vi "Process.vi"(9 "process sync":refnum<notifier>, 11 "DbgTimers in":refnum<class "DbgTimers.lvclass">) -> ()   [LabVIEW 2017, in "DbgTimers.lvclass"]
doc: "Developed by Kevin Thompson\nkevin@thompsonengineering.net\n\nCopyright 2018-2020\nThompson Engineering, LLC"
uses:
  DbgTimers.lvclass
  DataTypes/Read Data--cluster.ctl
  DataTypes/Process - AppData--cluster.ctl
  DataTypes/Settings--cluster.ctl
  DataTypes/Dependency--cluster.ctl
  DataTypes/Public Events--cluster.ctl
  Ichor_Common/DataTypes/TD Async CmdMsg EventData--cluster.ctl
  DbgTimers.lvclass/DbgTimers.ctl
  DataTypes/AsynMsg_DbgTimers--enum.ctl
  Accessors/Get Settings.vi
  Accessors/Get PublicEvents.vi
  Accessors/Get Dependency.vi
  Accessors/Get ObjData.vi
  Accessors/Set ObjData.vi
  <vilib>/TELLC/SMQ/Add States to Queue using MultiLine String with vData.vi
  Ichor_Common/Lib/ErrorHandler/ErrorHandler.lvclass
panel:
  out "LogFile path":path
  in  "Enable msTick Logging":bool
  out "DbgTimersReadData":T1
  in  "Exit":bool
  # "local data monitoring"
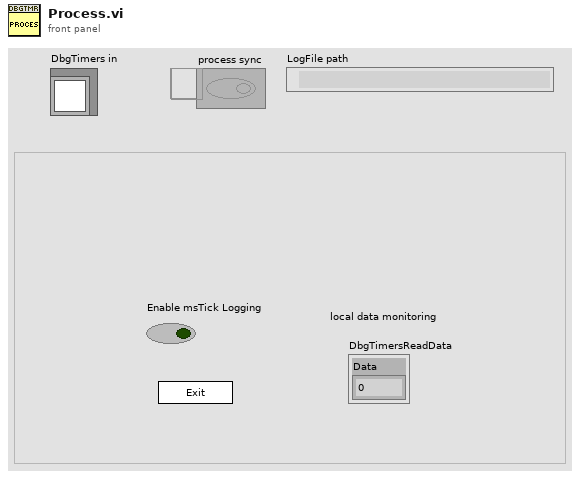
[diagram p1: front panel]
types:
  T1 = typedef "DbgTimers.lvclass/Read Data--cluster.ctl" = cluster{"Data":dbl}
  T2 = typedef "DbgTimers.lvclass/Process - AppData--cluster.ctl" = cluster{"Core":cluster{"Current VI Reference":refnum<vi>, "Close Panel on Exit?":bool}, "Your Boolean data":bool, "Your string data":string, "SMQ":refnum<queue>, "Initialized?":bool, "Self Reference":refnum<class "DbgTimers.lvclass">, "Simulation?":bool, "process sync":refnum<notifier>, "vData":variant, "Settings":T3, "Dependency":T4, "Public Events":T5, "msTickLogging?":bool}
  T3 = typedef "DbgTimers.lvclass/Settings--cluster.ctl" = cluster{"Simulation":bool, "DbgTimer LogFolder":path}
  T4 = typedef "DbgTimers.lvclass/Dependency--cluster.ctl" = cluster{"Config":refnum<class>, "ClassRef":refnum<class>}
  T5 = typedef "DbgTimers.lvclass/Public Events--cluster.ctl" = cluster{"DbgTimers.AsyncCmd Event":refnum<user-event>, "DbgTimers.AsyncMsg Event":refnum<user-event>, "stop process":refnum<user-event>}
  T6 = typedef "TELLC_Temp01.lvclass/Dependency--cluster.ctl" = cluster{"Config":refnum<class>, "ClassRef":refnum<class>}
  T7 = typedef "DbgTimers.lvclass/AsynMsg_DbgTimers--enum.ctl" = enum16{"DbgTimers.msTickLogEnabled"}
  T8 = enum32{"invalid app kind", "Development System", "Run Time System", "Student Edition", "Embedded LabVIEW", "Evaluation", "Custom"}
  T9 = enum32{"Invalid", "Standard", "Closed", "Hidden", "Minimized", "Maximized"}
  T10 = typedef "DbgTimers.lvclass/AsynCmd_DbgTimers--enum.ctl" = enum16{"DbgTimers.EnMsTickLogging", "DbgTimers.SetLogFolder"}
  T11 = typedef "DbgTimers.lvclass/ObjData--cluster.ctl" = cluster{"Settings":T3, "ReadData-placeholder":T1, "Timers":T12, "Enable msTick Logging":bool, "LogFile_msTickTimer":path}
  T12 = typedef "DbgTimers.lvclass/Timers--cluster.ctl" = cluster{"ms tick timers":T13[]}
  T13 = typedef "DbgTimers.lvclass/Millisecond Tick Timer--cluster.ctl" = cluster{"startTick":u32, "currentTick":u32, "elapsedTicks":u32, "totalElapsedTicks":u32}
  T14 = cluster{"Current VI Reference":refnum<vi>, "Close Panel on Exit?":bool}
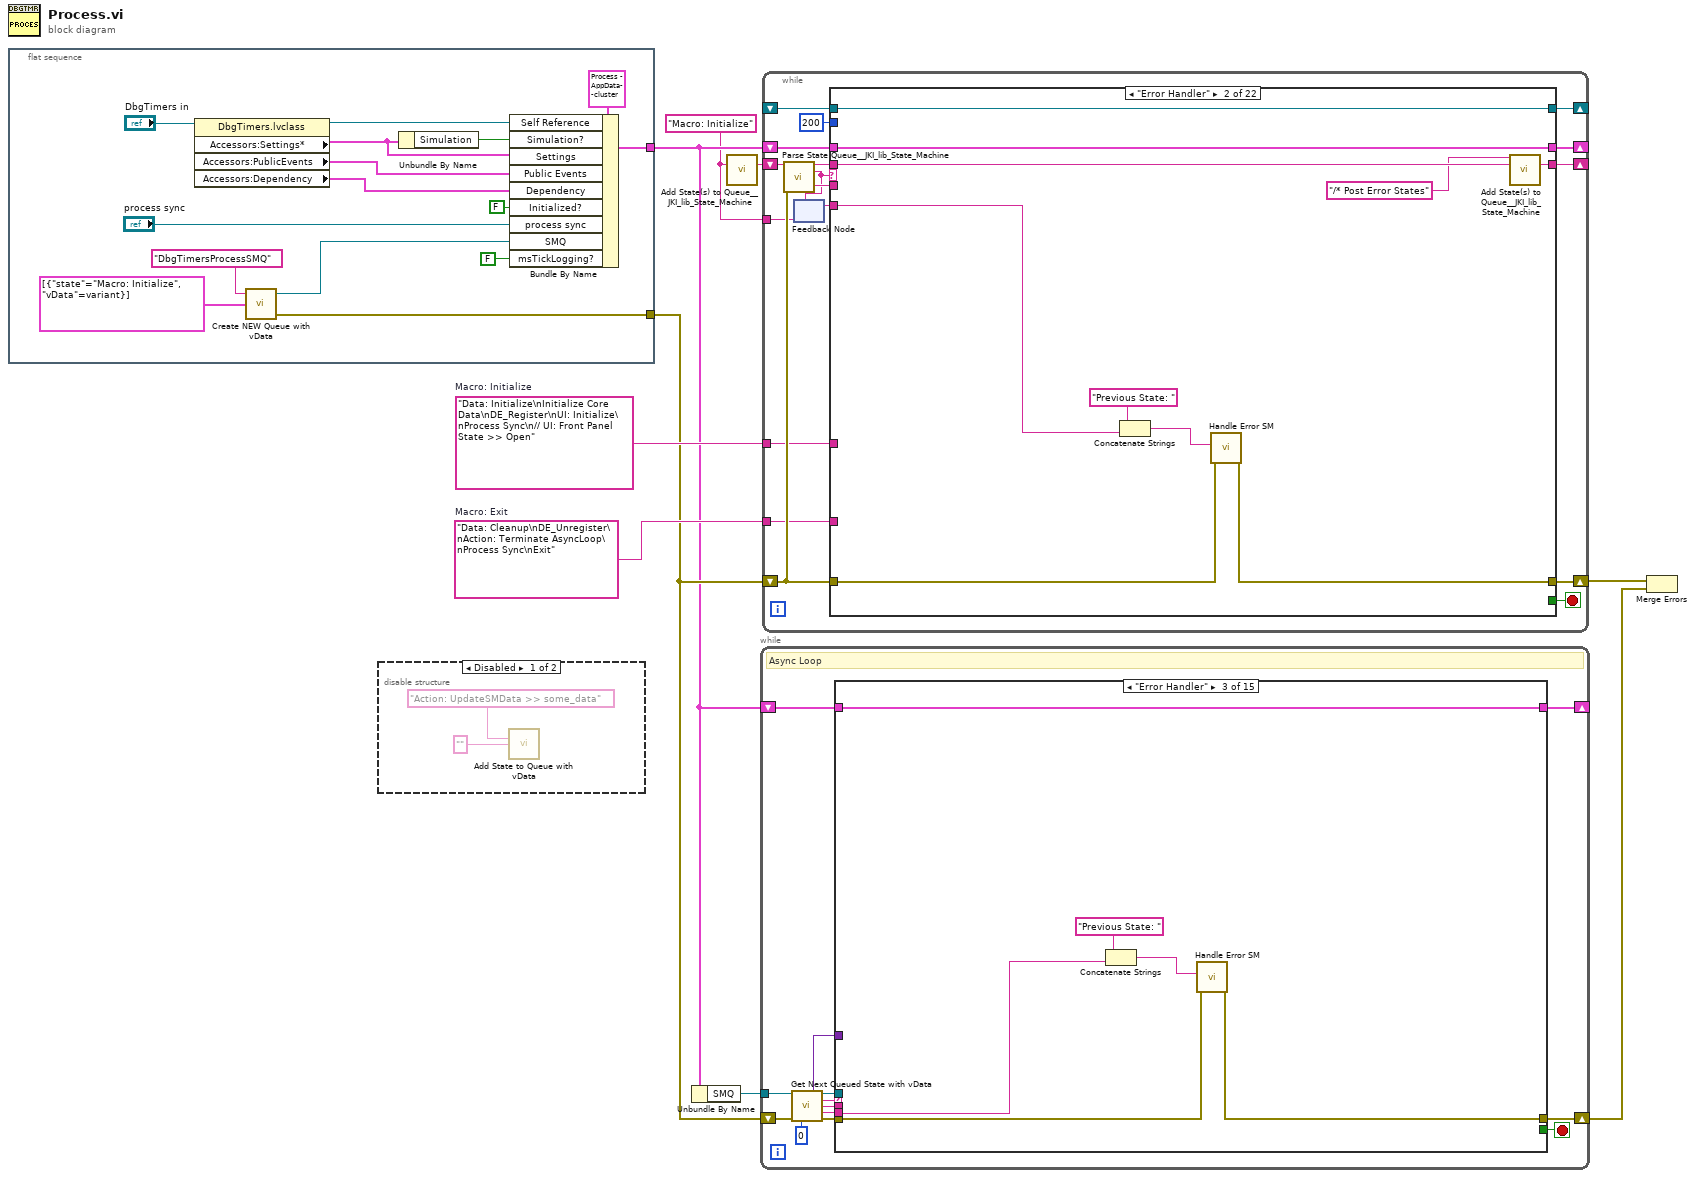
[diagram p0: block diagram]
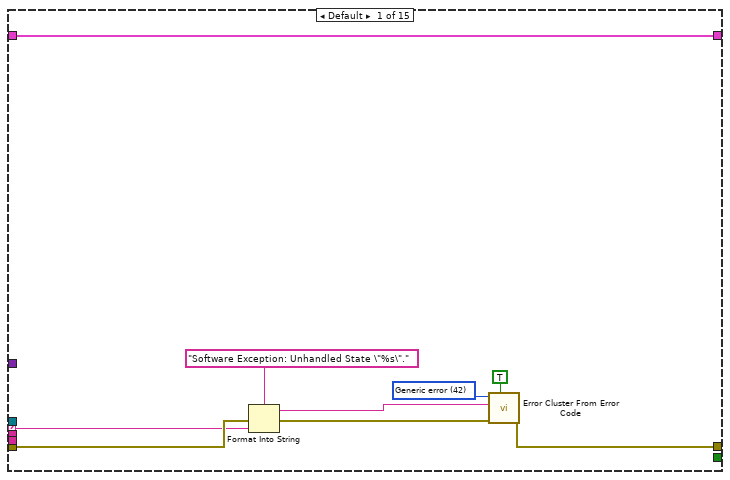
[diagram p3: hidden frame]
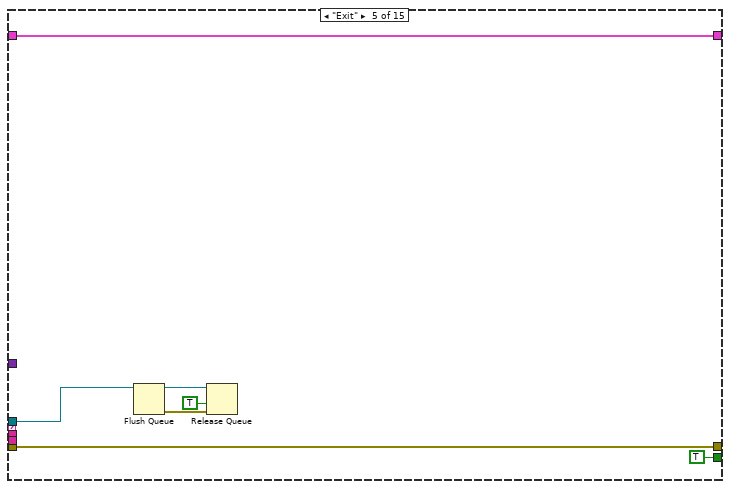
[diagram p6: hidden frame]
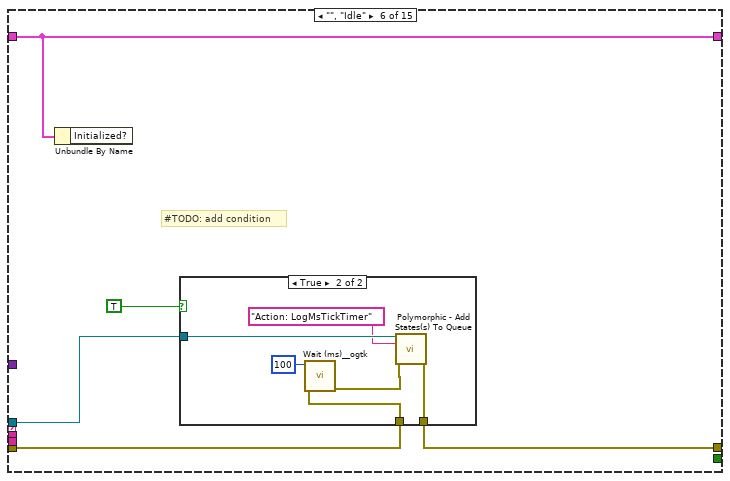
[diagram p7: hidden frame]
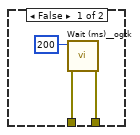
[diagram p8: hidden frame]
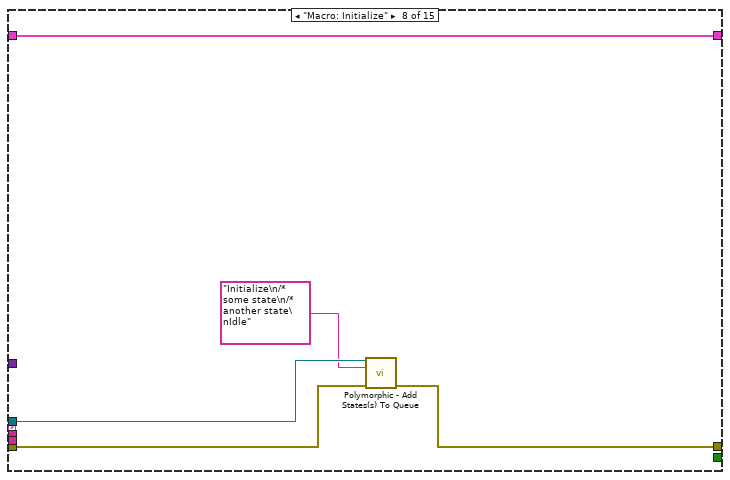
[diagram p10: hidden frame]
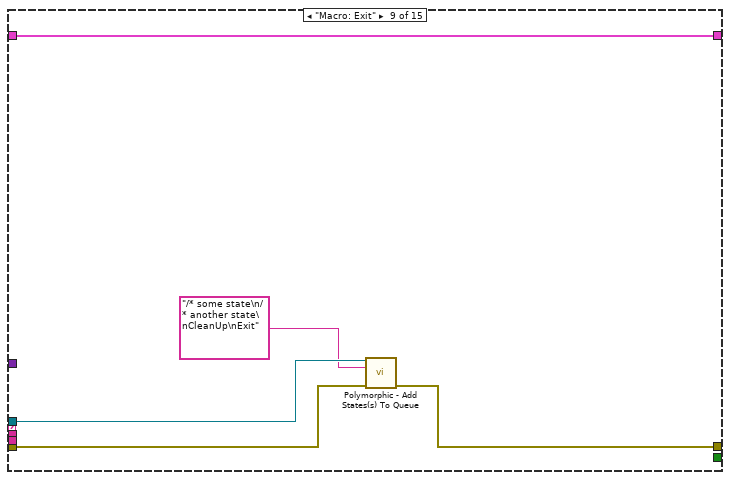
[diagram p11: hidden frame]
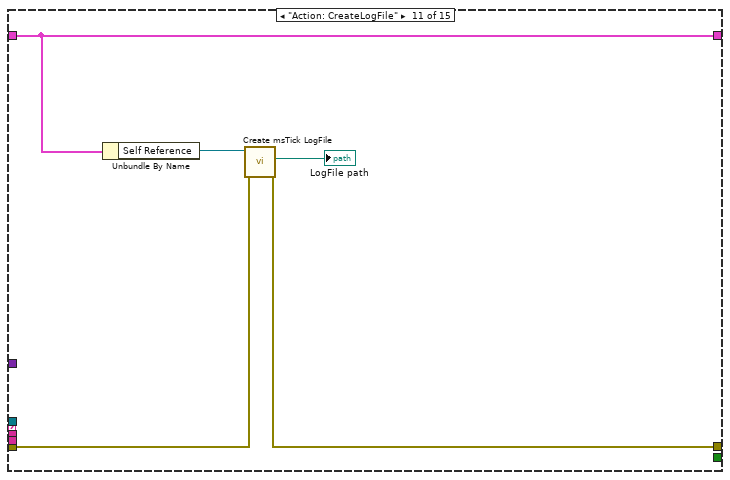
[diagram p13: hidden frame]
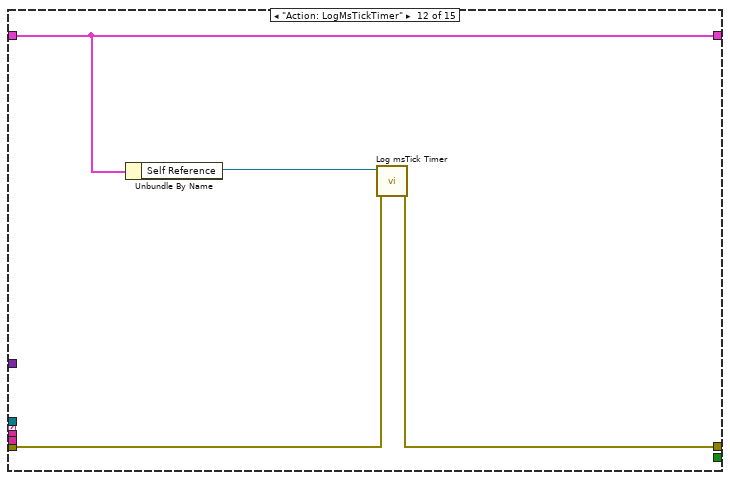
[diagram p14: hidden frame]
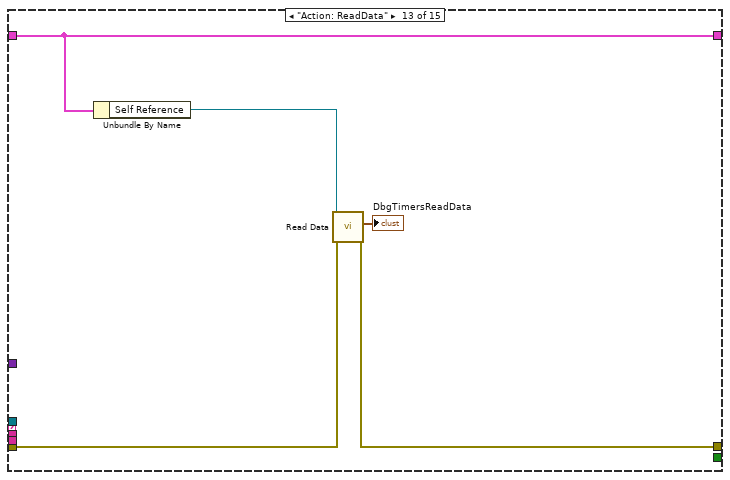
[diagram p15: hidden frame]
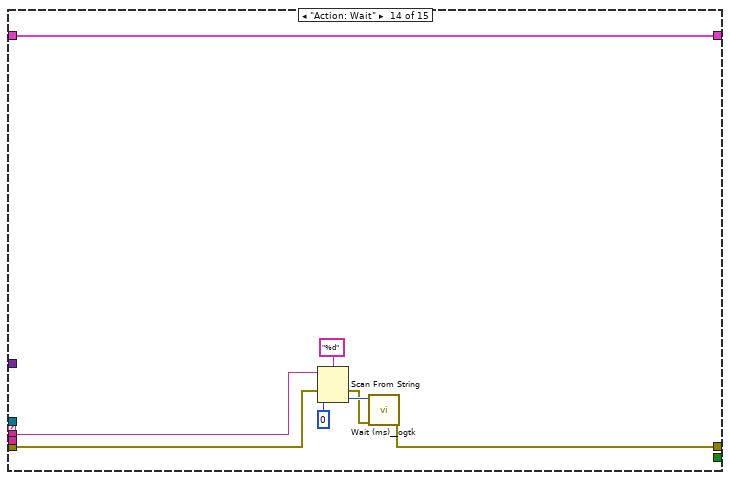
[diagram p16: hidden frame]
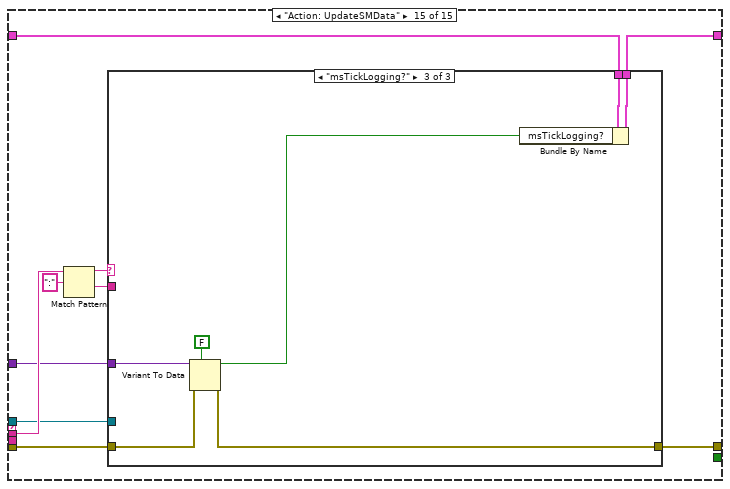
[diagram p17: hidden frame]
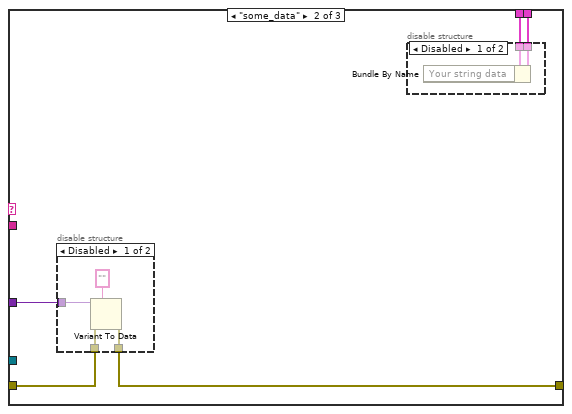
[diagram p19: hidden frame]
diagram:
  w7 = "Data: Cleanup\nDE_Unregister\nAction: Terminate AsyncLoop\nProcess Sync\nExit"  # Macro: Exit
  w8 = "Data: Initialize\nInitialize Core Data\nDE_Register\nUI: Initialize\nProcess Sync\n// UI: Front Panel State >> Open"  # Macro: Initialize
  w1 = "Macro: Initialize"
  n1 = flat-sequence {
    tunnel: [w24] -> w4
    tunnel: [w21] -> w6
    frame #0 {
      n2 = property class="DbgTimers.lvclass"(reference="DbgTimers in") -> (reference out=w17:refnum<class "DbgTimers.lvclass">, "Accessors:Settings*"=w12:T3, "Accessors:PublicEvents"=w14:T5, "Accessors:Dependency"=w15:T6)  [unwired: 1 in, 1 out]
      n3 = call <vilib>:"Create NEW Queue with vData.vi"("Initial States"=cluster{"state":string, "vData":variant}[] [{"state"="Macro: Initialize", "vData"=variant}], "Name (SMQ)"="DbgTimersProcessSMQ") -> ("error out"=w21:errorcluster, "queue out"=w23:refnum<queue>)  [unwired: 2 in]
      n4 = Unbundle By Name(w12) -> ("Simulation"=w13:bool)
      n5 = Bundle By Name(cluster=T2 {"Core"={"Current VI Reference"=refnum, "Close Panel on Exit?"=FALSE}, "Your Boolean data"=FALSE, "Your string data"="", "SMQ"=refnum, "Initialized?"=FALSE, "Self Reference"=refnum, "Simulation?"=FALSE, "process sync"=refnum, "vData"=variant, "Settings"={"Simulation"=FALSE, "DbgTimer LogFolder"=path ""}, "Dependency"={"Config"=refnum, "ClassRef"=refnum}, "Public Events"={"DbgTimers.AsyncCmd Event"=refnum, "DbgTimers.AsyncMsg Event"=refnum, "stop process"=refnum}, "msTickLogging?"=FALSE} ("SM2 AppData"), "Self Reference"=w17, "Simulation?"=w13, "Settings"=w12, "Public Events"=w14, "Dependency"=w15, "Initialized?"=FALSE, "process sync"="process sync", "SMQ"=w23, "msTickLogging?"=FALSE) -> (w24:T2)
    }
  }
  n6 = disable-structure shown="Disabled" {
    frame Disabled {
      n7 = call <vilib>:"Add State to Queue with vData.vi"("state in"="Action: UpdateSMData >> some_data", "vData (\"\")"="") -> ()  [unwired: 10 in, 4 out]
    }
    frame Enabled {
    }
  }
  n8 = Unbundle By Name(w4) -> ("SMQ"=w5:refnum<queue>)
  n9 = call <vilib>:"Add State(s) to Queue__JKI_lib_State_Machine.vi"("State(s) in (\"\")"=w1) -> ("States Out"=w9:string)  [unwired: 14 in]
  n10 = while {
    shift-right: [w36] -> w2
    shift-left: w6 -> [w38]
    tunnel: w5 -> [w34]
    shift-right: [w32] -> _
    shift-left: w4 -> [w33]
    stop <- w27 stop-if-true
    # "Async Loop"
    n11 = call <vilib>:"Get Next Queued State with vData.vi"("queue in"=w34, "error in (no error)"=w38, "timeout (100)"=0) -> ("vData out"=w31:variant, "queue out"=w35:refnum<queue>, "Next State"=w39:string, "queued msg"=w29:string, "Prev State"=w28:string, "error out"=w37:errorcluster)  [unwired: 6 in, 1 out]
    n12 = case shown="\"Error Handler\"" w39 {
      tunnel: w35 -> [_ _ _ _ w59 w67 _ w85 w90 _ _ _ _ _ w121]
      tunnel: w29 -> [_ _ _ _ _ _ _ _ _ _ _ _ _ w110 w123]
      selector: w39 -> [w40 _ _ _ _ _ _ _ _ _ _ _ _ _ _]
      tunnel: w37 -> [w42 w50 w53 w58 w65 w70 w81 w84 w89 w93 w96 w100 w105 w109 w118]
      tunnel: [w41 w50 w52 w58 w65 w69 w81 w83 w88 w93 w95 w99 w104 w112 w117] -> w36
      tunnel: w33 -> [w48 w49 w56 w57 w64 w66 w80 w86 w91 w92 w98 w102 w107 w115 w120]
      tunnel: [w48 w49 w56 w57 w64 w66 w80 w86 w91 w92 w98 w102 w107 w115 w119] -> w32
      tunnel: w31 -> [_ _ _ _ _ _ _ _ _ _ _ _ _ _ w122]
      tunnel: w28 -> [_ _ w51 _ _ _ _ _ _ _ _ _ _ _ _]
      tunnel: [_ _ _ _ TRUE _ _ _ _ _ _ _ _ _ _] -> w27
      frame Default {
        w44 = 42 items=["No error", "Argument error", "Memory is full", "Out of zone", "End of file", "File already open", "Generic file I/O error", "File not found", "File permission error", "Disk is full", "Duplicate path", "Too many files open", "System feature not enabled", "Resource file not found", "Cannot add resource", "Resource not found", "Image not found", "Image memory error", "Pen does not exist", "Config type invalid", "Config token not found", "Config parse error", "Config memory error", "Bad external code format", "Bad external code offset", "External code not present", "Null window", "Destroy window error", "Null menu", "Print aborted", "Bad print record", "Print driver error", "Windows error during printing", "Memory error during printing", "Print dialog error", "Generic print error", "Invalid device refnum", "Device not found", "Device parameter error", "Device unit error", "Cannot open device", "Device call aborted", "Generic error", "Cancelled by user", "Object ID too low", "Object ID too high", "Object not in heap", "Unknown heap", "Unknown object (invalid DefProc)", "Unknown object (DefProc not in table)", "Message out of range", "Invalid (null) method", "Unknown message", "Manager call not supported", "Bad address", "Network operation in progress", "Network operation timed out", "Connection is busy", "Network attribute not supported", "Network error", "Address in use", "System out of memory", "Connection aborted", "Connection refused", "Not connected", "Already connected", "Connection closed", "Initialization error (interapplication manager)", "Bad occurrence", "Wait on unbound occurrence handler", "Occurrence queue overflow", "Datalog type conflict", "Unused", "Unrecognized type (interapplication manager)", "Memory corrupt", "Failed to make temporary DLL", "Old CIN version", "Drag socket not found", "Failed to load drop-object", "Failed to register OLE object", "Failed to release OLE object", "Format specifier type mismatch", "Unknown format specifier", "Too few format specifiers", "Too many format specifiers", "Scan failed", "Newer CIN version", "Error converting to variant", "Runtime menu error", "Password tampered", "Variant attribute not found", "Incompatible variant data type", "Event data is not available", "Event Store is not present", "Occurrence is not found", "Event Queue is not created", "Event info is not available", "Refnum passed is NULL", "Error retrieving Class GUID", "Error retrieving CoClass GUID", "Error retrieving TypeLib GUID.", "Bad built application magic bytes.", "Specific driver is different from the specific driver associated with the Logical Name.", "There is no session opened to the class driver.", "Max Error", "MAX - Error with config objects", "MAX - Error loading configuration", "MAX - Group not supported"]
        n13 = Format Into String(format string="Software Exception: Unhandled State \"%s\"." ("message"), error in=w42, w40) -> (resulting string=w45:string, error out=w46:errorcluster)  [unwired: 1 in]
        n14 = call <vilib>:"Error Cluster From Error Code.vi"("show call chain? (False)"=TRUE, "error in (no error)"=w46, "error message (\"\")"=w45, "error code (0)"=w44) -> ("error out"=w41:errorcluster)  [unwired: 5 in]
      }
      frame "Initialize" {
      }
      frame "Error Handler" {
        n15 = Concatenate Strings("Previous State: ", w51) -> (w54:string)
        n16 = call "Handle Error SM.vi"("error in (no error)"=w53, "CustomMessage"=w54) -> ("error out"=w52:errorcluster)  [unwired: 7 in, 2 out]
      }
      frame "CleanUp" {
      }
      frame "Exit" {
        n17 = Flush Queue(queue=w59) -> (queue out=w62:refnum<queue>, error out=w61:errorcluster)  [unwired: 1 in, 1 out]
        n18 = Release Queue(queue=w62, force destroy? (F)=TRUE, error in (no error)=w61) -> ()  [unwired: 3 out]
      }
      frame "", "Idle" {
        # "#TODO: add condition"
        n19 = Unbundle By Name(w66) -> ()  [unwired: 1 out]
        n20 = case shown="True" TRUE {
          tunnel: w70 -> [w73 w75]
          tunnel: [w72 w79] -> w69
          tunnel: w67 -> [_ w78]
          frame False {
            n21 = call <userlib>:"Wait (ms)__ogtk.vi"("error in (no error)"=w73, "milliseconds to wait"=u32 200) -> ("error out"=w72:errorcluster)  [unwired: 8 in, 1 out]
          }
          frame True {
            n22 = call <userlib>:"Wait (ms)__ogtk.vi"("error in (no error)"=w75, "milliseconds to wait"=u32 100) -> ("error out"=w76:errorcluster)  [unwired: 8 in, 1 out]
            n23 = call-poly <vilib>:"Polymorphic - Add States(s) To Queue.vi"("queue in"=w78, "state in"="Action: LogMsTickTimer", "error in"=w76) -> ("error out"=w79:errorcluster)  [unwired: 9 in, 3 out]
          }
        }
      }
      frame "------ Macro ------" {
      }
      frame "Macro: Initialize" {
        n24 = call-poly <vilib>:"Polymorphic - Add States(s) To Queue.vi"("queue in"=w85, "states in"="Initialize\n/* some state\n/* another state\nIdle", "error in"=w84) -> ("error out"=w83:errorcluster)  [unwired: 10 in, 2 out]
      }
      frame "Macro: Exit" {
        n25 = call-poly <vilib>:"Polymorphic - Add States(s) To Queue.vi"("queue in"=w90, "states in"="/* some state\n/* another state\nCleanUp\nExit", "error in"=w89) -> ("error out"=w88:errorcluster)  [unwired: 10 in, 2 out]
      }
      frame "------ Action ------" {
      }
      frame "Action: CreateLogFile" {
        n26 = Unbundle By Name(w98) -> ("Self Reference"=w97:refnum<class "DbgTimers.lvclass">)
        n27 = call "Create msTick LogFile.vi"("error in (no error)"=w96, "DbgTimers in"=w97) -> ("error out"=w95:errorcluster, "LogFile path"=→"LogFile path":path)  [unwired: 7 in, 1 out]
      }
      frame "Action: LogMsTickTimer" {
        n28 = Unbundle By Name(w102) -> ("Self Reference"=w101:refnum<class "DbgTimers.lvclass">)
        n29 = call "Log msTick Timer.vi"("error in (no error)"=w100, "DbgTimers in"=w101) -> ("error out"=w99:errorcluster)  [unwired: 7 in, 2 out]
      }
      frame "Action: ReadData" {
        n30 = Unbundle By Name(w107) -> ("Self Reference"=w106:refnum<class "DbgTimers.lvclass">)
        n31 = call "Read Data.vi"("error in (no error)"=w105, "DbgTimers in"=w106) -> ("error out"=w104:errorcluster, "DbgTimersReadData"=→"DbgTimersReadData":T1)  [unwired: 7 in, 1 out]
      }
      frame "Action: Wait" {
        n32 = Scan From String(format string="%d", input string=w110, error in=w109, default 1=u32 0) -> (error out=w108:errorcluster, output 1=w114:u32)  [unwired: 1 in, 2 out]
        n33 = call <userlib>:"Wait (ms)__ogtk.vi"("error in (no error)"=w108, "milliseconds to wait"=w114) -> ("error out"=w112:errorcluster)  [unwired: 8 in, 1 out]
      }
      frame "Action: UpdateSMData" {
        n34 = Match Pattern(string=w123, regular expression=":") -> (before substring=w125:string, after substring=w116:string)  [unwired: 1 in, 2 out]
        n35 = case shown="\"msTickLogging?\"" w125 {
          tunnel: w122 -> [_ w132 w147]
          tunnel: w121 -> [_ _ _]
          tunnel: w120 -> [w126 w131 w146]
          tunnel: [w126 w130 w145] -> w119
          tunnel: w118 -> [w127 w129 w144]
          tunnel: [w127 w128 w143] -> w117
          tunnel: w116 -> [_ _ _]
          frame Default {
            # "#NOTE:\noptionally add error here."
          }
          frame "some_data" {
            n36 = disable-structure shown="Disabled" {
              disable-tunnel: w132 -> [w139 _]
              disable-tunnel: w129 -> [w137 w140]
              disable-tunnel: [w136 w140] -> w128
              frame Disabled {
                n37 = Variant To Data(error in=w137, type="", Variant=w139) -> (error out=w136:errorcluster)  [unwired: 1 out]
              }
              frame Enabled {
              }
            }
            n38 = disable-structure shown="Disabled" {
              disable-tunnel: w131 -> [w134 w135]
              disable-tunnel: [w133 w135] -> w130
              frame Disabled {
                n39 = Bundle By Name(cluster=w134) -> (w133:T2)  [unwired: 1 in]
              }
              frame Enabled {
              }
            }
          }
          frame "msTickLogging?" {
            n40 = Variant To Data(error in=w144, type=FALSE, Variant=w147) -> (data=w141:bool, error out=w143:errorcluster)
            n41 = Bundle By Name(cluster=w146, "msTickLogging?"=w141) -> (w145:T2)
          }
        }
      }
    }
  }
  n42 = while {
    shift-right: [w158] -> _
    shift-left: w4 -> [w157]
    shift-right: [w161] -> w3
    shift-left: w6 -> [w156]
    shift-right: [w160] -> _
    shift-left: w9 -> [w162]
    shift-right: [w155] -> _
    shift-left: _ -> [w154]
    tunnel: w8 -> [w152]
    tunnel: w7 -> [w151]
    tunnel: w1 -> [w150]
    stop <- w159 stop-if-true
    n43 = call <vilib>:"Parse State Queue__JKI_lib_State_Machine.vi"("State Queue"=w162, "Error In (no error)"=w156) -> ("Remaining States"=w164:string, "Current State"=w149:string, "Arguments"=w163:string)  [unwired: 11 in]
    n44 = feedback #1(w150) -> (w148:string)
    n45 = feedback-in #1(w149) -> ()
    n46 = case shown="\"Error Handler\"" w149 {
      selector: w149 -> [w166 _ _ _ _ _ _ _ _ _ _ _ _ _ _ _ _ _ _ _ _ _]
      tunnel: w164 -> [w170 w186 w192 w200 w308 w321 w329 w334 w338 w343 w359 w366 w371 w379 w388 w400 w427 w433 w444 w449 w460 w469]
      tunnel: w163 -> [_ _ _ _ _ _ _ _ _ _ _ _ _ _ w383 w394 _ _ _ _ w450 _]
      tunnel: w157 -> [w168 w184 w190 w198 w305 w312 w326 w331 w337 w340 w347 w361 w368 w374 w386 w396 w424 w430 w441 w446 w458 w466]
      tunnel: [w172 w177 w189 w197 w306 w318 w322 w332 w335 w341 w346 w362 w369 w375 w384 w397 w425 w431 w442 w447 w451 w461] -> w161
      tunnel: w156 -> [w171 w178 w189 w196 w306 w318 w323 _ w335 w341 _ w363 w369 w376 w385 w398 w425 w431 w442 w447 w452 w462]
      tunnel: [w169 w185 w191 w199 w307 w320 w328 w334 w338 w342 w358 w365 w370 w378 w387 w399 w426 w432 w443 w448 w459 w468] -> w160
      tunnel: [_ _ TRUE _ _ _ _ _ _ _ _ _ _ _ _ _ _ _ _ _ _ _] -> w159
      tunnel: [w168 w184 w190 w195 w305 w319 w326 w331 w337 w340 w354 w361 w368 w374 w386 w396 w424 w430 w441 w446 w458 w466] -> w158
      tunnel: [w165 w182 w187 w193 w304 w309 w327 w333 w336 w339 w353 w360 w367 w377 w382 w393 w423 w429 w435 w445 w457 w467] -> w155
      tunnel: w154 -> [w165 w182 w187 w193 w304 w309 w327 _ w336 w339 w353 w360 w367 w377 w382 w393 w423 w429 w435 w445 w457 w467]
      tunnel: 200 ("Timeout") -> [_ _ _ w194 _ _ _ _ _ _ _ _ _ _ _ _ _ _ _ _ _ _]
      tunnel: w152 -> [_ _ _ _ _ _ _ _ _ _ _ _ _ _ _ _ _ w428 _ _ _ _]
      tunnel: w151 -> [_ _ _ _ _ _ _ _ _ _ _ _ _ _ _ _ _ _ w434 _ _ _]
      tunnel: w148 -> [_ w179 _ _ _ _ _ _ _ _ _ _ _ _ _ _ _ _ _ _ _ _]
      frame Default {
        w175 = 42 items=["No error", "Argument error", "Memory is full", "Out of zone", "End of file", "File already open", "Generic file I/O error", "File not found", "File permission error", "Disk is full", "Duplicate path", "Too many files open", "System feature not enabled", "Resource file not found", "Cannot add resource", "Resource not found", "Image not found", "Image memory error", "Pen does not exist", "Config type invalid", "Config token not found", "Config parse error", "Config memory error", "Bad external code format", "Bad external code offset", "External code not present", "Null window", "Destroy window error", "Null menu", "Print aborted", "Bad print record", "Print driver error", "Windows error during printing", "Memory error during printing", "Print dialog error", "Generic print error", "Invalid device refnum", "Device not found", "Device parameter error", "Device unit error", "Cannot open device", "Device call aborted", "Generic error", "Cancelled by user", "Object ID too low", "Object ID too high", "Object not in heap", "Unknown heap", "Unknown object (invalid DefProc)", "Unknown object (DefProc not in table)", "Message out of range", "Invalid (null) method", "Unknown message", "Manager call not supported", "Bad address", "Network operation in progress", "Network operation timed out", "Connection is busy", "Network attribute not supported", "Network error", "Address in use", "System out of memory", "Connection aborted", "Connection refused", "Not connected", "Already connected", "Connection closed", "Initialization error (interapplication manager)", "Bad occurrence", "Wait on unbound occurrence handler", "Occurrence queue overflow", "Datalog type conflict", "Unused", "Unrecognized type (interapplication manager)", "Memory corrupt", "Failed to make temporary DLL", "Old CIN version", "Drag socket not found", "Failed to load drop-object", "Failed to register OLE object", "Failed to release OLE object", "Format specifier type mismatch", "Unknown format specifier", "Too few format specifiers", "Too many format specifiers", "Scan failed", "Newer CIN version", "Error converting to variant", "Runtime menu error", "Password tampered", "Variant attribute not found", "Incompatible variant data type", "Event data is not available", "Event Store is not present", "Occurrence is not found", "Event Queue is not created", "Event info is not available", "Refnum passed is NULL", "Error retrieving Class GUID", "Error retrieving CoClass GUID", "Error retrieving TypeLib GUID.", "Bad built application magic bytes.", "Specific driver is different from the specific driver associated with the Logical Name.", "There is no session opened to the class driver.", "Max Error", "MAX - Error with config objects", "MAX - Error loading configuration", "MAX - Group not supported"]
        # "Current State"
        n47 = Format Into String(format string="Software Exception: Unhandled State \"%s\"." ("message"), error in=w171, w166) -> (resulting string=w174:string, error out=w173:errorcluster)  [unwired: 1 in]
        n48 = call <vilib>:"Error Cluster From Error Code.vi"("show call chain? (False)"=TRUE, "error in (no error)"=w173, "error message (\"\")"=w174, "error code (0)"=w175) -> ("error out"=w172:errorcluster)  [unwired: 5 in]
        n49 = call <vilib>:"Add State(s) to Queue__JKI_lib_State_Machine.vi"("State(s) in (\"\")"=w170) -> ("States Out"=w169:string)  [unwired: 14 in]
      }
      frame "Error Handler" {
        n50 = Concatenate Strings("Previous State: ", w179) -> (w181:string)
        n51 = call "Handle Error SM.vi"("error in (no error)"=w178, "CustomMessage"=w181) -> ("error out"=w177:errorcluster)  [unwired: 7 in, 2 out]
        n52 = call <vilib>:"Add State(s) to Queue__JKI_lib_State_Machine.vi"("State(s) in Front (\"\")"="/* Post Error States", "State(s) in (\"\")"=w186) -> ("States Out"=w185:string)  [unwired: 13 in]
      }
      frame "Exit" {
        n53 = call <vilib>:"Add State(s) to Queue__JKI_lib_State_Machine.vi"("State(s) in (\"\")"=w192) -> ("States Out"=w191:string)  [unwired: 14 in]
      }
      frame "", "Event Structure", "Idle" {
        n54 = event shown="[6] \"Enable msTick Logging\": Value Change" {
          selector: w193 -> [_ _ _ _ _ _ _]
          dyn-events: _ -> [_ _ _ _ _ _ _]
          timeout: w194 -> [_ _ _ _ _ _ _]
          tunnel: w200 -> [w204 w209 w215 w218 w225 w242 w303]
          tunnel: [w203 w208 w214 w217 w224 w241 w303] -> w199
          tunnel: w198 -> [w201 w206 w212 w220 w228 w231 w293]
          tunnel: [w202 w207 w213 w221 w229 w239 w287] -> w197
          tunnel: w196 -> [w202 w207 w213 w221 w229 w238 w295]
          tunnel: [w201 w206 w212 w220 w227 w233 w296] -> w195
          event Timeout {
            n55 = event-data() -> ()  [unwired: 1 in, 1 out]
            n56 = call <vilib>:"Add State(s) to Queue__JKI_lib_State_Machine.vi"("State(s) in (\"\")"=w204) -> ("States Out"=w203:string)  [unwired: 14 in]
          }
          event "Exit": Value Change {
            n57 = event-data() -> ()  [unwired: 1 in, 1 out]
            n58 = call <vilib>:"Add State(s) to Queue__JKI_lib_State_Machine.vi"("State(s) in Front (\"\")"="Macro: Exit", "State(s) in (\"\")"=w209) -> ("States Out"=w208:string)  [unwired: 13 in]
          }
          event Panel Close? {
            n59 = event-data() -> ()  [unwired: 1 in, 1 out]
            n60 = event-data("Discard?"=TRUE) -> ()  [unwired: 1 in, 1 out]
            n61 = call <vilib>:"Add State(s) to Queue__JKI_lib_State_Machine.vi"("State(s) in Front (\"\")"="Macro: Exit", "State(s) in (\"\")"=w215) -> ("States Out"=w214:string)  [unwired: 13 in]
          }
          event Menu Selection (User) {
            n62 = event-data() -> ("ItemTag"=w219:string)  [unwired: 1 in, 2 out]
            n63 = case shown="\"False\", Default" w219 {
              tunnel: [""] -> w216
              frame "False", Default {
              }
            }
            n64 = call <vilib>:"Add State(s) to Queue__JKI_lib_State_Machine.vi"("State(s) in Front (\"\")"=w216, "State(s) in (\"\")"=w218) -> ("States Out"=w217:string)  [unwired: 13 in]
          }
          event User Event {
            n65 = event-data() -> ("notifier out"=w226:refnum<notifier>)  [unwired: 1 in]
            n66 = Bundle By Name(cluster=w228, "process sync"=w226) -> (w227:T2)
            n67 = call <vilib>:"Add State(s) to Queue__JKI_lib_State_Machine.vi"("State(s) in Front (\"\")"="Macro: Exit", "State(s) in (\"\")"=w225) -> ("States Out"=w224:string)  [unwired: 13 in]
          }
          event User Event {
            n68 = event-data() -> ("CmdMsg"=w236:string, "vData"=w240:variant)  [unwired: 1 in, 1 out]
            n69 = Unbundle By Name(w231) -> ("Self Reference"=w232:refnum<class "DbgTimers.lvclass">)
            n70 = Unbundle By Name(w231) -> ("SMQ"=w230:refnum<queue>)
            n71 = call "get async cmd.vi"("error in (no error)"=w238, "Cmd String in"=w236) -> ("error out"=w237:errorcluster, "AsyncCmd"=w235:T10)  [unwired: 8 in]
            n72 = case shown="\"DbgTimers.SetLogFolder\"" w235 {
              tunnel: w240 -> [_ w272 w283]
              tunnel: w237 -> [w248 w271 w284]
              tunnel: [w247 w250 w276] -> w239
              tunnel: [_ "" _] -> w234
              tunnel: w231 -> [w243 w269 w273]
              tunnel: [w243 w268 w273] -> w233
              tunnel: w232 -> [_ w257 w281]
              tunnel: w231 -> [_ _ _]
              tunnel: w230 -> [_ w256 _]
              frame Default {
                n73 = call <vilib>:"Build Error Cluster_ModKT .vi"("Prepend String (\"\")"="Invalid Async Cmd" ("Prepend String (\"\")"), "code"=42, "error? (F)"=TRUE, "error in (no error)"=w248) -> ("error out"=w247:errorcluster)  [unwired: 3 in, 1 out]
              }
              frame "DbgTimers.EnMsTickLogging" {
                n74 = property class="DbgTimers.lvclass"(reference=w257) -> (reference out=w263:refnum<class "DbgTimers.lvclass">, error out=w260:errorcluster, "Accessors:ObjData*"=w262:T11)  [unwired: 1 in]
                n75 = Variant To Data(error in=w271, type=FALSE, Variant=w272) -> (data=w255:bool, error out=w251:errorcluster)
                n76 = Bundle By Name(cluster=w262, "Enable msTick Logging"=w255) -> (w261:T11)
                n77 = call <vilib>:"Add State to Queue with vData.vi"("queue in"=w256, "state in"="Action: UpdateSMData >> msTickLogging", "vData (\"\")"=w255) -> ("queue out"=w265:refnum<queue>, "error out"=w264:errorcluster)  [unwired: 9 in, 2 out]
                n78 = property class="DbgTimers.lvclass"(reference=w263, error in=w260, "Accessors:ObjData*"=w261) -> (reference out=w253:refnum<class "DbgTimers.lvclass">, error out=w252:errorcluster)
                n79 = Not(x=w255) -> (.not. x?=w266:bool)
                n80 = call <vilib>:"Add State to Queue with vData.vi"("queue in"=w265, "state in"="Action: CreateLogFile", "bypass (F)"=w266, "error in"=w264) -> ()  [unwired: 8 in, 4 out]
                n81 = Bundle By Name(cluster=w269, "msTickLogging?"=w255) -> (w268:T2)
                n82 = call "Generate Async Msg Event.vi"("error in (no error)"=w252, "vData"=w255, "AsyncMsg"=AsynMsg_DbgTimers--enum."DbgTimers.msTickLogEnabled", "DbgTimers in"=w253) -> ("error out"=w249:errorcluster)  [unwired: 6 in, 1 out]
                n83 = Merge Errors(w249, w251) -> (w250:errorcluster)
              }
              frame "DbgTimers.SetLogFolder" {
                n84 = property class="DbgTimers.lvclass"(reference=w281) -> (reference out=w280:refnum<class "DbgTimers.lvclass">, "Accessors:ObjData*"=w279:T11)  [unwired: 1 in, 1 out]
                n85 = Variant To Data(error in=w284, type=path "", Variant=w283) -> (data=w277:path, error out=w275:errorcluster)
                n86 = Bundle By Name(cluster=w279, "Settings.DbgTimer LogFolder"=w277) -> (w278:T11)
                n87 = property class="DbgTimers.lvclass"(reference=w280, "Accessors:ObjData*"=w278) -> (error out=w274:errorcluster)  [unwired: 1 in, 1 out]
                n88 = Merge Errors(w274, w275) -> (w276:errorcluster)
              }
            }
            n89 = call <vilib>:"Add State(s) to Queue__JKI_lib_State_Machine.vi"("State(s) in Front (\"\")"=w234, "State(s) in (\"\")"=w242) -> ("States Out"=w241:string)  [unwired: 13 in]
          }
          event "Enable msTick Logging": Value Change {
            n90 = event-data() -> ("NewVal"=w285:bool)  [unwired: 1 in]
            n91 = Unbundle By Name(w293) -> ("Self Reference"=w292:refnum<class "DbgTimers.lvclass">)
            n92 = Unbundle By Name(w293) -> ("SMQ"=w299:refnum<queue>)
            n93 = property class="DbgTimers.lvclass"(reference=w292) -> (reference out=w291:refnum<class "DbgTimers.lvclass">, error out=w288:errorcluster, "Accessors:ObjData*"=w290:T11)  [unwired: 1 in]
            n94 = call <vilib>:"Add State to Queue with vData.vi"("queue in"=w299, "state in"="Action: UpdateSMData >> msTickLogging", "vData (\"\")"=w285, "error in"=w295) -> ("queue out"=w298:refnum<queue>, "error out"=w297:errorcluster)  [unwired: 8 in, 2 out]
            n95 = Bundle By Name(cluster=w290, "Enable msTick Logging"=w285) -> (w289:T11)
            n96 = Not(x=w285) -> (.not. x?=w301:bool)
            n97 = call <vilib>:"Add State to Queue with vData.vi"("queue in"=w298, "state in"="Action: CreateLogFile", "bypass (F)"=w301, "error in"=w297) -> ("error out"=w294:errorcluster)  [unwired: 8 in, 3 out]
            n98 = property class="DbgTimers.lvclass"(reference=w291, error in=w288, "Accessors:ObjData*"=w289) -> (error out=w286:errorcluster)  [unwired: 1 out]
            n99 = Bundle By Name(cluster=w293, "msTickLogging?"=w285) -> (w296:T2)
            n100 = Merge Errors(w286, w294) -> (w287:errorcluster)
          }
        }
      }
      frame "---------- Core ----------" {
        n101 = call <vilib>:"Add State(s) to Queue__JKI_lib_State_Machine.vi"("State(s) in (\"\")"=w308) -> ("States Out"=w307:string)  [unwired: 14 in]
      }
      frame "Initialize Core Data" {
        # "originally closed?"
        # "exe?"
        n102 = property class="VI"() -> ("Front Panel.Open"=w317:bool)  [unwired: 2 in, 2 out]
        n103 = property class="App"() -> ("App.Kind"=w316:T8)  [unwired: 2 in, 2 out]
        n104 = control-ref of="Current VI Reference"() -> (w310:refnum<vi>)
        n105 = Not(x=w317) -> (.not. x?=w314:bool)
        n106 = Equal?(x=w316, y=T8."Run Time System" ("Application:Kind")) -> (x = y?=w313:bool)
        n107 = Or(x=w314, y=w313) -> (x .or. y?=w311:bool)
        n108 = Bundle By Name(cluster=w312, "Core.Current VI Reference"=w310, "Core.Close Panel on Exit?"=w311) -> (w319:T2)
        n109 = call <vilib>:"Add State(s) to Queue__JKI_lib_State_Machine.vi"("State(s) in (\"\")"=w321) -> ("States Out"=w320:string)  [unwired: 14 in]
      }
      frame "Process Sync" {
        n110 = Unbundle By Name(w326) -> ("process sync"=w325:refnum<notifier>)
        n111 = Send Notification(notification=TRUE, notifier=w325, error in (no error)=w323) -> (error out=w322:errorcluster)  [unwired: 1 out]
        n112 = call <vilib>:"Add State(s) to Queue__JKI_lib_State_Machine.vi"("State(s) in (\"\")"=w329) -> ("States Out"=w328:string)  [unwired: 14 in]
      }
      frame "DE_Register" {
        n113 = Unbundle By Name(w331) -> ("Public Events"=w330:T5)
        n114 = register-events(w330) -> (reference out=w333:refnum<event-registration>, error out=w332:errorcluster)  [unwired: 2 in]
      }
      frame "DE_Unregister" {
        n115 = Unregister For Events(event registration refnum=w336, error in=w335) -> ()  [unwired: 1 out]
      }
      frame "---------- Data ----------" {
        n116 = call <vilib>:"Add State(s) to Queue__JKI_lib_State_Machine.vi"("State(s) in (\"\")"=w343) -> ("States Out"=w342:string)  [unwired: 14 in]
      }
      frame "Data: Initialize" {
        w355 = T14 {"Current VI Reference"=refnum, "Close Panel on Exit?"=FALSE}  # Core
        w357 = TRUE  # Your Boolean data
        w356 = ""  # Your string data
        n117 = Unbundle By Name(w347) -> ("Self Reference"=w352:refnum<class "DbgTimers.lvclass">)
        n118 = property class="DbgTimers.lvclass"(reference=w352) -> (reference out=w351:refnum<class "DbgTimers.lvclass">, error out=w348:errorcluster, "Accessors:ObjData*"=w350:T11)  [unwired: 1 in]
        n119 = Bundle By Name(cluster=w350, "Enable msTick Logging"=FALSE, "LogFile_msTickTimer"=path "") -> (w349:T11)
        n120 = Bundle By Name(cluster=w347, "Core"=w355, "Your Boolean data"=w357, "Your string data"=w356) -> (w354:T2)
        n121 = property class="DbgTimers.lvclass"(reference=w351, error in=w348, "Accessors:ObjData*"=w349) -> (error out=w346:errorcluster)  [unwired: 1 out]
        n122 = call <vilib>:"Add State(s) to Queue__JKI_lib_State_Machine.vi"("State(s) in (\"\")"=w359) -> ("States Out"=w358:string)  [unwired: 14 in]
      }
      frame "Data: Cleanup" {
        n123 = Unbundle By Name(w361) -> ("Core.Current VI Reference"=w364:refnum<vi>)
        n124 = Close Reference(reference=w364, error in (no error)=w363) -> (error out=w362:errorcluster)
        n125 = call <vilib>:"Add State(s) to Queue__JKI_lib_State_Machine.vi"("State(s) in (\"\")"=w366) -> ("States Out"=w365:string)  [unwired: 14 in]
      }
      frame "---------- UI ----------" {
        n126 = call <vilib>:"Add State(s) to Queue__JKI_lib_State_Machine.vi"("State(s) in (\"\")"=w371) -> ("States Out"=w370:string)  [unwired: 14 in]
      }
      frame "UI: Initialize" {
        n127 = Unbundle By Name(w374) -> ("Core.Current VI Reference"=w373:refnum<vi>)
        n128 = call <userlib>:"Fit VI window to Largest Dec__ogtk.vi"("error in (no error)"=w376, "VI Ref (calling VI)"=w373) -> ("error out"=w375:errorcluster, "dup VI Ref"=w372:refnum<vi>)  [unwired: 4 in]
        n129 = disable-structure shown="Disabled" {
          disable-tunnel: w372 -> [w381 _]
          frame Disabled {
            n130 = property class="VI"(reference=w381, "Front Panel.Title"="*VI Title*" ("Front Panel Window:Title")) -> ()  [unwired: 1 in, 2 out]
          }
          frame Enabled {
          }
        }
        n131 = call <vilib>:"Add State(s) to Queue__JKI_lib_State_Machine.vi"("State(s) in (\"\")"=w379) -> ("States Out"=w378:string)  [unwired: 14 in]
      }
      frame "UI: Cursor Set" {
        # "Argument"
        n132 = case shown="\"Idle\", Default" w383 {
          tunnel: w385 -> [w390 w392]
          tunnel: [w389 w391] -> w384
          frame "Idle", Default {
            n133 = call <vilib>:"Unset Busy.vi"("error in (no error)"=w390) -> ("error out"=w389:errorcluster)  [unwired: 10 in]
          }
          frame "Busy" {
            n134 = call <vilib>:"Set Busy.vi"("error in (no error)"=w392) -> ("error out"=w391:errorcluster)  [unwired: 9 in, 1 out]
          }
        }
        n135 = call <vilib>:"Add State(s) to Queue__JKI_lib_State_Machine.vi"("State(s) in (\"\")"=w388) -> ("States Out"=w387:string)  [unwired: 14 in]
      }
      frame "UI: Front Panel State" {
        # "Argument"
        n136 = Unbundle By Name(w396) -> ("Core.Current VI Reference"=w395:refnum<vi>)
        n137 = case shown="\"Close\"" w394 {
          tunnel: w398 -> [w404 w417]
          tunnel: [w406 w418] -> w397
          tunnel: w395 -> [w405 w415]
          frame "Open", Default {
            n138 = property class="VI"(reference=w405, error in=w404) -> (reference out=w402:refnum<vi>, error out=w403:errorcluster, "Front Panel.Open"=w401:bool)
            n139 = case shown="False" w401 {
              tunnel: [w409 w412] -> w406
              tunnel: w403 -> [w408 w412]
              tunnel: w402 -> [w407 _]
              frame False {
                n140 = invoke class="VI" method="FP.Open"(reference=w407, error in=w408, "Activate"=TRUE, "State"=T9."Standard") -> (error out=w409:errorcluster)  [unwired: 1 in, 4 out]
              }
              frame True {
              }
            }
          }
          frame "Close" {
            n141 = property class="VI"(reference=w415, error in=w417) -> (reference out=w414:refnum<vi>, error out=w416:errorcluster, "Front Panel.Open"=w413:bool)
            n142 = case shown="True" w413 {
              tunnel: [w419 w422] -> w418
              tunnel: w416 -> [w419 w421]
              tunnel: w414 -> [_ w420]
              frame False {
              }
              frame True {
                n143 = invoke class="VI" method="FP.Close"(reference=w420, error in=w421) -> (error out=w422:errorcluster)  [unwired: 1 in, 2 out]
              }
            }
          }
        }
        n144 = call <vilib>:"Add State(s) to Queue__JKI_lib_State_Machine.vi"("State(s) in (\"\")"=w400) -> ("States Out"=w399:string)  [unwired: 14 in]
      }
      frame "---------- Macro ----------" {
        n145 = call <vilib>:"Add State(s) to Queue__JKI_lib_State_Machine.vi"("State(s) in (\"\")"=w427) -> ("States Out"=w426:string)  [unwired: 14 in]
      }
      frame "Macro: Initialize" {
        n146 = call <vilib>:"Add State(s) to Queue__JKI_lib_State_Machine.vi"("State(s) in Front (\"\")"=w428, "State(s) in (\"\")"=w433) -> ("States Out"=w432:string)  [unwired: 13 in]
      }
      frame "Macro: Exit" {
        n147 = Unbundle By Name(w441) -> ("Core.Close Panel on Exit?"=w440:bool)
        n148 = Select(t="UI: Front Panel State >> Close", s=w440, f="") -> (s? t:f=w437:string)
        n149 = call <vilib>:"Add State(s) to Queue__JKI_lib_State_Machine.vi"("State(s) in (\"\")"=w437, "State(s) at Back (\"\")"=w434) -> ("States Out"=w436:string)  [unwired: 13 in]
        n150 = call <vilib>:"Add State(s) to Queue__JKI_lib_State_Machine.vi"("State(s) in Front (\"\")"=w436, "State(s) in (\"\")"=w444) -> ("States Out"=w443:string)  [unwired: 13 in]
      }
      frame "---------- Action ----------" {
        n151 = call <vilib>:"Add State(s) to Queue__JKI_lib_State_Machine.vi"("State(s) in (\"\")"=w449) -> ("States Out"=w448:string)  [unwired: 14 in]
      }
      frame "Action: Wait" {
        n152 = Scan From String(format string="%d", input string=w450, error in=w452, default 1=u32 0) -> (error out=w456:errorcluster, output 1=w455:u32)  [unwired: 1 in, 2 out]
        n153 = call <userlib>:"Wait (ms)__ogtk.vi"("error in (no error)"=w456, "milliseconds to wait"=w455) -> ("error out"=w451:errorcluster)  [unwired: 8 in, 1 out]
        n154 = call <vilib>:"Add State(s) to Queue__JKI_lib_State_Machine.vi"("State(s) in (\"\")"=w460) -> ("States Out"=w459:string)  [unwired: 14 in]
      }
      frame "Action: Terminate AsyncLoop" {
        n155 = Unbundle By Name(w466) -> ("SMQ"=w465:refnum<queue>)
        n156 = Flush Queue(queue=w465) -> (queue out=w464:refnum<queue>)  [unwired: 1 in, 2 out]
        n157 = call <vilib>:"Add State to Queue with vData.vi"("queue in"=w464, "state in"="Macro: Exit", "error in"=w462) -> ("error out"=w461:errorcluster)  [unwired: 9 in, 3 out]
        n158 = call <vilib>:"Add State(s) to Queue__JKI_lib_State_Machine.vi"("State(s) in (\"\")"=w469) -> ("States Out"=w468:string)  [unwired: 14 in]
      }
    }
  }
  n159 = Merge Errors(w3, w2) -> ()  [unwired: 1 out]
